vi "Pack Mutexed Publish Request.vi"(4 "PublicationPolicy":refnum<class "IPublicationPolicy.lvclass">, 6 "Return Error Transport":refnum<class "ITransport.lvclass">, 7 "Publisher ID":string, 8 "error in (no error)":errorcluster, 9 "Publish Time (Use Current Time)":timestamp, 10 "Datum Value or Type":variant, 11 "Datum Name":string) -> (0 "error out":errorcluster, 3 "MutexedPublishRequest Out":refnum<class "MutexedPublishRequest.lvclass">)   [LabVIEW 2020, in "IMediator.lvlib" / "MutexedPublishRequest.lvclass"]
uses:
  <vilib>/gpm_packages/@cs/mva-core/Source/IMediator/MutexedPublishRequest/MutexedPublishRequest.lvclass
  C:/Program Files/National Instruments/LabVIEW 2020/vi.lib/gpm_packages/@cs/mva-core/Source/IMediator/PublishRequest/PublishRequest.lvclass
  <vilib>/gpm_packages/@cs/mva-core/Source/IMediator/IPublicationPolicy/IPublicationPolicy.lvclass
  <vilib>/gpm_packages/@cs/transport/Source/ITransport/ITransport.lvclass
  <vilib>/gpm_packages/@cs/mva-core/Source/IMediator/PublishRequest/PublishRequest.lvclass/PublishRequest.ctl
  <vilib>/gpm_packages/@cs/mva-core/Source/IMediator/MutexedPublishRequest/MutexedPublishRequest.lvclass/MutexedPublishRequest.ctl
  <vilib>/Utility/error.llb/Error Cluster From Error Code.vi
  <vilib>/gpm_packages/@cs/mva-core/Source/IMediator/PublishRequest/PublishRequest.lvclass
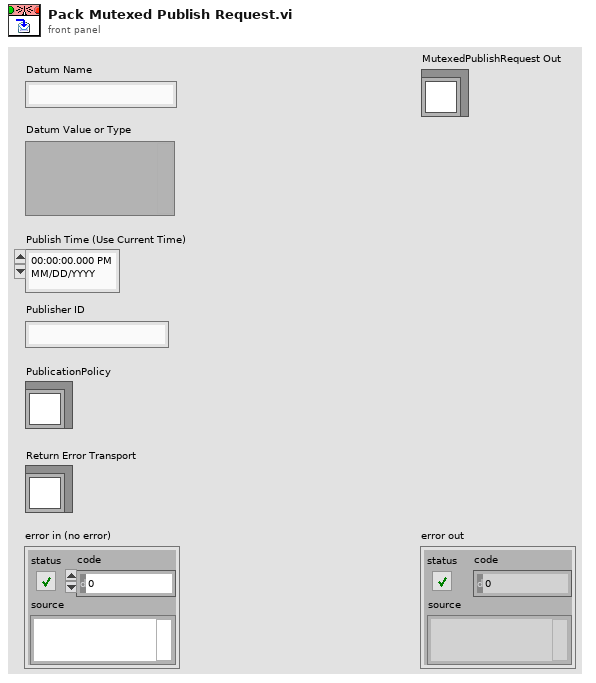
[diagram p1: front panel]
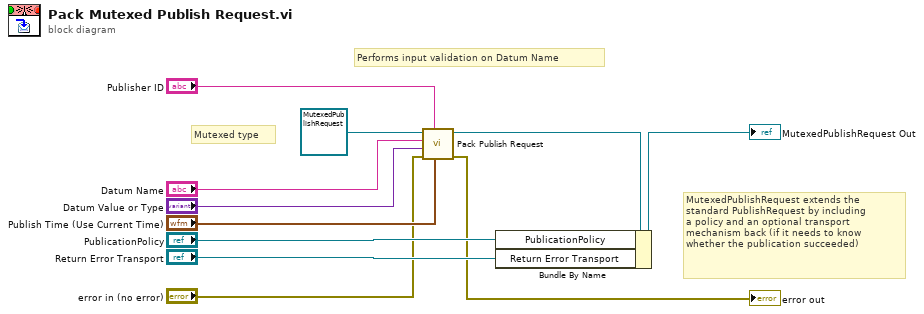
[diagram p0: block diagram]
diagram:
  # "Mutexed type"
  # "Performs input validation on Datum Name"
  # "MutexedPublishRequest extends the\nstandard PublishRequest by including\na policy and an optional transport\nmechanism back (if it needs to know\nwhether the publication succeeded)"
  n1 = call <vilib>:"Pack Publish Request.vi"("Publication Time (Use Current Time)"="Publish Time (Use Current Time)", "Publisher ID"="Publisher ID", "error in (no error)"="error in (no error)", "Value"="Datum Value or Type", "Datum Name"="Datum Name", "PublishRequest In"=refnum<class "MutexedPublishRequest.lvclass"> refnum ("PublishRequest in")) -> ("error out"=→"error out":errorcluster, "PublishRequest Out"=w8:refnum<class "MutexedPublishRequest.lvclass">)  [unwired: 4 in]
  n2 = Bundle By Name(cluster=w8, "PublicationPolicy"="PublicationPolicy", "Return Error Transport"="Return Error Transport") -> (→"MutexedPublishRequest Out":refnum<class "MutexedPublishRequest.lvclass">)
